vi "Detect Devices.vi"(8 "error in (no error)":errorcluster, 11 "VISA resource name":refnum<visa-resource-name>) -> (0 "error out":errorcluster, 2 "Connected Devices and Axes":string[](array[string]), 3 "VISA resource name out":refnum<visa-resource-name>)   [LabVIEW 2013, in "Zaber A Series.lvlib"]
doc: "Polls the connected devices and returns an array of the Connected Devices and Axes. Elements of the array can be used as an input for the Device and Axis input of other VIs in this library, for example through a dropdown list.\n\nThis VI requires that the Initialize VI has been called with the same serial port."
uses:
  Zaber A Series.lvlib
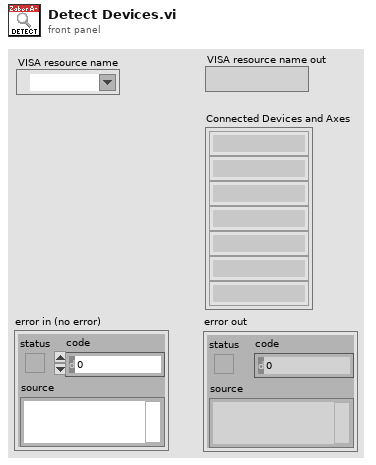
[diagram p1: front panel]
types:
  T1 = cluster{"Device":string, "Axis":string, "Reply Flag":string, "Status":string, "Warning Flags":string, "Data":string}[]
  T2 = cluster{"Device":string, "Axis":string, "Reply Flag":string, "Status":string, "Warning Flags":string, "Data":string}
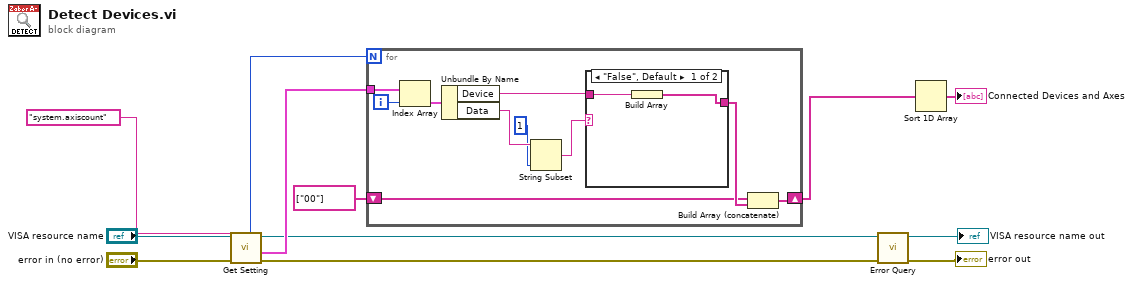
[diagram p0: block diagram]
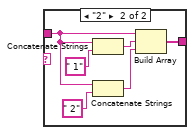
[diagram p2: hidden frame]
diagram:
  n1 = call "Get Setting.vi"("error in (no error)"="error in (no error)", "Setting"="system.axiscount" ("Common Settings"), "VISA resource name"="VISA resource name") -> ("error out"=w3:errorcluster, "Response Bundle Array"=w6:T1, "VISA resource name out"=w4:refnum<visa-resource-name>, "Number of Replies"=w5:i32)  [unwired: 4 in, 1 out]
  n2 = for {
    N: w5 -> [_]
    tunnel: w6 -> [w22]
    shift-right: [w14] -> w10
    shift-left: string[] ["00"] -> [w13]
    i -> [w15]
    n3 = Index Array(array=w22, index=w15) -> (element=w21:T2)
    n4 = Unbundle By Name(w21) -> ("Device"=w20:string, "Data"=w18:string)
    n5 = String Subset(string=w18, length (rest)=1 ("length (rest)")) -> (substring=w16:string)  [unwired: 1 in]
    n6 = case shown="\"False\", Default" w16 {
      tunnel: w20 -> [w24 w25]
      tunnel: [w23 w27] -> w19
      frame "False", Default {
        n7 = Build Array(w24) -> (w23:string[])
      }
      frame "2" {
        n8 = Concatenate Strings(w25, " 1" ("string")) -> (w26:string)
        n9 = Concatenate Strings(w25, " 2" ("string")) -> (w28:string)
        n10 = Build Array(w25, w26, w28) -> (w27:string[])
      }
    }
    n11 = Build Array (concatenate)(w13, w19) -> (w14:string[])
  }
  n12 = call "Error Query.vi"("error in (no error)"=w3, "VISA resource name"=w4) -> ("error out"=→"error out":errorcluster, "VISA resource name out"=→"VISA resource name out":refnum<visa-resource-name>)  [unwired: 6 in, 2 out]
  n13 = Sort 1D Array(array=w10) -> (sorted array=→"Connected Devices and Axes":string[])
